vi "Basic LabVIEW OPC UA Client-Read.vi"() -> ()   [LabVIEW 2020]
uses:
  <vilib>/OPCUA/NI OPC UA Client.lvlib
  <vilib>/OPCUA/client/Multiple Read Double.vi
  <vilib>/OPCUA/NI OPC UA Utility.lvlib
panel:
  in  "Item Path":string="Nodes.Temperature"
  in  "Stop Button":bool
  out "Temperature Value":dbl=23.0
  in  "Server Endpoint URL":string="opc.tcp://XPS15HPH:49580"
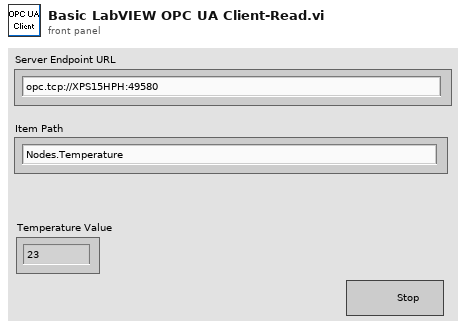
[diagram p1: front panel]
types:
  T1 = cluster{"message mode":enum16{"None", "Sign", "Sign and Encrypt"}, "security":enum16{"Basic256", "Basic128Rsa15"}}
  T2 = typedef "OPC UA Client Refnum.ctl" = refnum<k21>
  T3 = typedef "NodeId.ctl" = string
  T4 = typedef "OPC UA StatusCode.ctl" = u32
  T5 = cluster{"node ID":T3, "value ":dbl, "timestamp":timestamp, "status":T4}[]
  T6 = cluster{"node ID":T3, "value ":dbl, "timestamp":timestamp, "status":T4}
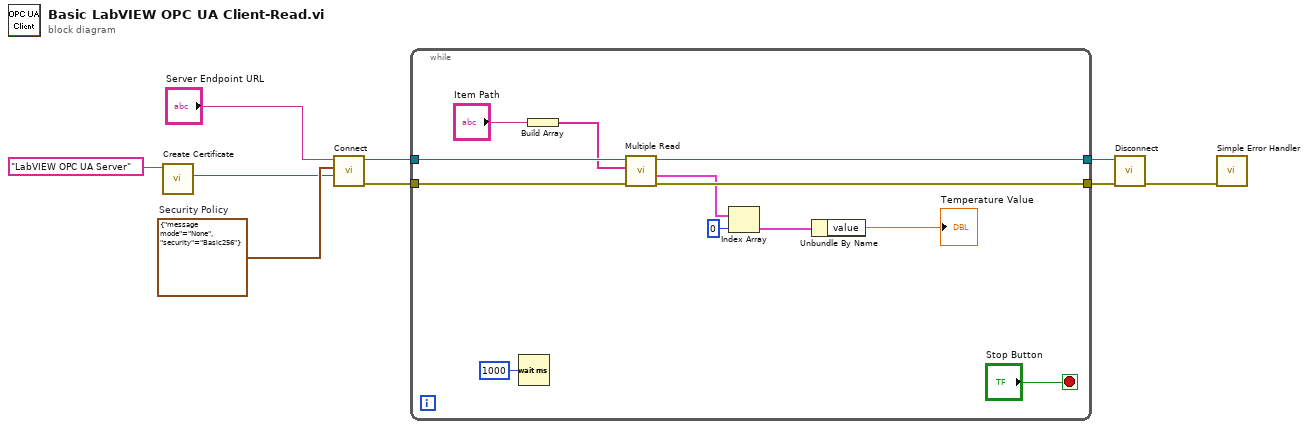
[diagram p0: block diagram]
diagram:
  w3 = T1 {"message mode"=enum."None", "security"=enum."Basic256"}  # Security Policy
  n1 = call <vilib>:"Create Certificate.vi"("certificate name in"="LabVIEW OPC UA Server") -> ("certificate path"=w1:path)  [unwired: 7 in, 3 out]
  n2 = call <vilib>:"Connect.vi"("client certificate file"=w1, "security policy"=w3, "server endpoint URL"="Server Endpoint URL") -> ("error out"=w8:errorcluster, "OPC UA client refnum out"=w9:T2)  [unwired: 6 in, 1 out]
  n3 = while {
    tunnel: w9 -> [w19]
    tunnel: w8 -> [w18]
    tunnel: [w17] -> w7
    tunnel: [w16] -> w5
    stop <- "Stop Button" stop-if-true
    n4 = Wait (ms)(milliseconds to wait=u32 1000) -> ()  [unwired: 1 out]
    n5 = Build Array "Build Array"("Item Path") -> (w15:string[])
    n6 = call-poly <vilib>:"Multiple Read.vi"("error in (no error)"=w18, "node IDs"=w15, "OPC UA client refnum in"=w19) -> ("error out"=w16:errorcluster, "results"=w13:T5, "OPC UA client refnum out"=w17:T2)  [unwired: 5 in, 1 out]
    n7 = Index Array "Index Array"(array=w13, index=0) -> (element=w11:T6)
    n8 = Unbundle By Name "Unbundle By Name"(w11) -> ("value"=→"Temperature Value":dbl)
  }
  n9 = call <vilib>:"Disconnect.vi"("error in (no error)"=w5, "OPC UA client refnum in"=w7) -> ("error out"=w6:errorcluster)  [unwired: 9 in]
  n10 = call <vilib>:"Simple Error Handler.vi"("error in (no error)"=w6) -> ()  [unwired: 4 in, 5 out]
